vi "Success Box.vi"(8 "error in":errorcluster) -> (0 "error out":errorcluster)   [LabVIEW 2015]
uses:
  <vilib>/Platform/browser.llb/Open URL in Default Browser (string).vi
  <vilib>/Utility/cursorutil.llb/Set Cursor (Icon Pict).vi
panel:
  in  "Link":bool
  in  "OK":bool
  # "Program operation completed successfully. For more details\nand usage examples, visit the TI support wiki at:"
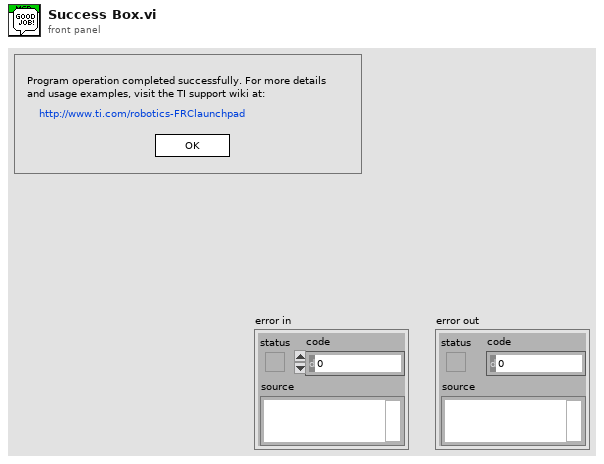
[diagram p1: front panel]
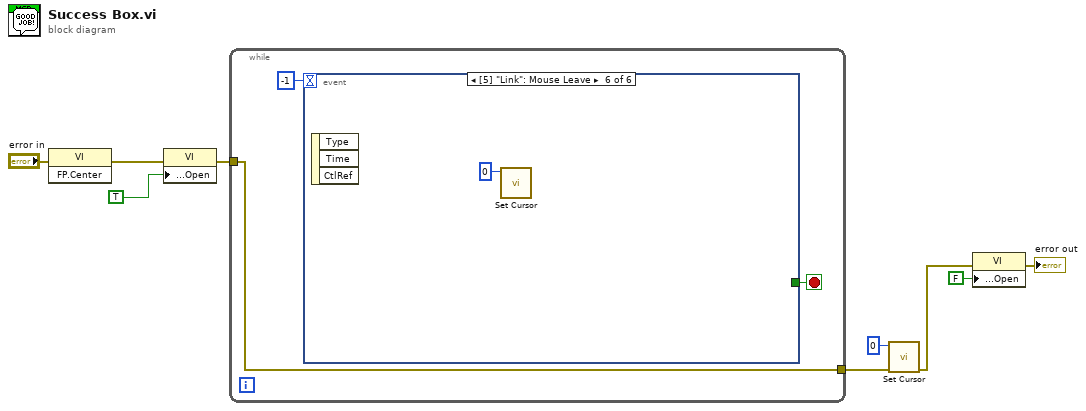
[diagram p0: block diagram]
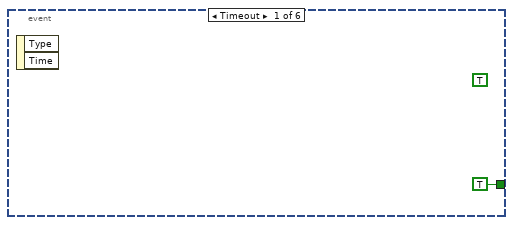
[diagram p2: hidden frame]
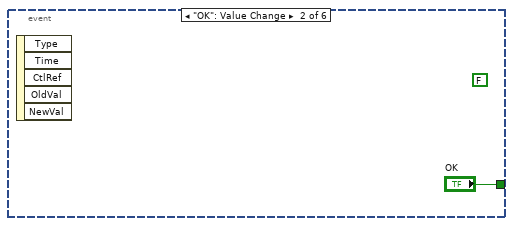
[diagram p3: hidden frame]
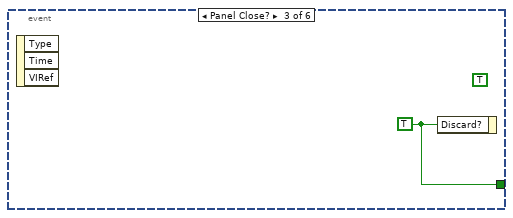
[diagram p4: hidden frame]
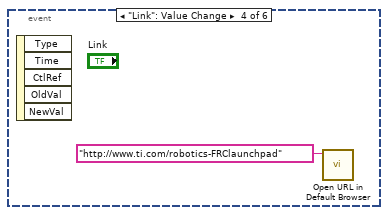
[diagram p5: hidden frame]
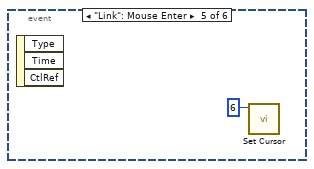
[diagram p6: hidden frame]
diagram:
  n1 = invoke class="VI" method="FP.Center"(error in="error in") -> (error out=w8:errorcluster)  [unwired: 2 in, 2 out]
  n2 = property class="VI"(error in=w8, "Front Panel Window:Open"=TRUE) -> (error out=w7:errorcluster)  [unwired: 1 in, 1 out]
  n3 = while {
    tunnel: w7 -> [w10]
    tunnel: [w10] -> w2
    stop <- w11 stop-if-true
    n4 = event shown="[5] \"Link\": Mouse Leave" {
      selector: _ -> [_ _ _ _ _ _]
      dyn-events: _ -> [_ _ _ _ _ _]
      timeout: -1 -> [_ _ _ _ _ _]
      tunnel: [TRUE ("Cancel") "OK" w15 _ _ _] -> w11
      event Timeout {
        (unwired) TRUE
        n5 = event-data() -> ()  [unwired: 1 in, 2 out]
      }
      event "OK": Value Change {
        (unwired) FALSE
        n6 = event-data() -> ()  [unwired: 1 in, 5 out]
      }
      event Panel Close? {
        w15 = TRUE ("Discard?")
        (unwired) TRUE
        n7 = event-data() -> ()  [unwired: 1 in, 3 out]
        n8 = event-data("Discard?"=w15) -> ()  [unwired: 1 in, 1 out]
      }
      event "Link": Value Change {
        n9 = event-data() -> ()  [unwired: 1 in, 5 out]
        n10 = call-poly <vilib>:"Open URL in Default Browser.vi"("URL"="http://www.ti.com/robotics-FRClaunchpad") -> ()  [unwired: 5 in, 2 out]
      }
      event "Link": Mouse Enter {
        n11 = event-data() -> ()  [unwired: 1 in, 3 out]
        n12 = call-poly <vilib>:"Set Cursor.vi"("icon"=u16 6) -> ()  [unwired: 9 in, 2 out]
      }
      event "Link": Mouse Leave {
        n13 = event-data() -> ()  [unwired: 1 in, 3 out]
        n14 = call-poly <vilib>:"Set Cursor.vi"("icon"=u16 0) -> ()  [unwired: 9 in, 2 out]
      }
    }
  }
  n15 = call-poly <vilib>:"Set Cursor.vi"("error in (no error)"=w2, "icon"=u16 0) -> ("error out"=w1:errorcluster)  [unwired: 8 in, 1 out]
  n16 = property class="VI"(error in=w1, "Front Panel Window:Open"=FALSE) -> (error out=→"error out":errorcluster)  [unwired: 1 in, 1 out]
